vi "Result Info Schema Show FP.vi"(8 "error in (no error)":errorcluster, 10 "Test Log":refnum<vi>, 11 "Result Info in":refnum<class "Result Info.lvclass">) -> (0 "error out":errorcluster, 3 "Result Info out":refnum<class "Result Info.lvclass">)   [LabVIEW 2023]
uses:
  Result Info.lvclass
  D:/eDCU LTT/VT LTT Project/Source Code/Data Analysis/Subpanel-Abstract/Subpanel-Abstract.lvclass
  C:/Program Files/National Instruments/LabVIEW 2023/vi.lib/ActorFramework/Actor/Actor.lvclass
  D:/eDCU LTT/VT LTT Project/Source Code/Data Analysis/Result Info/Result Info/Result Info.lvclass
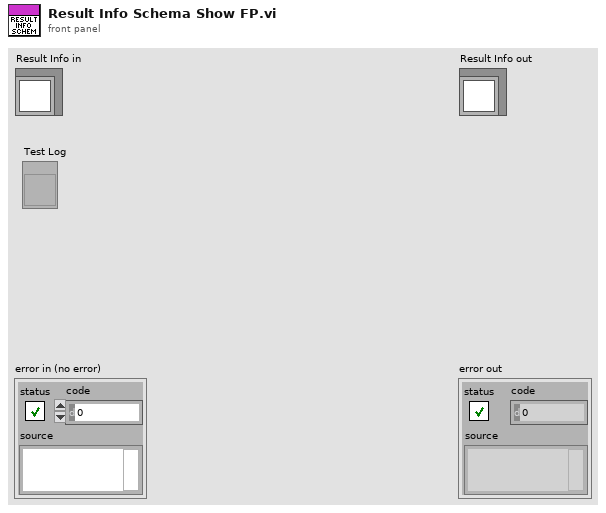
[diagram p1: front panel]
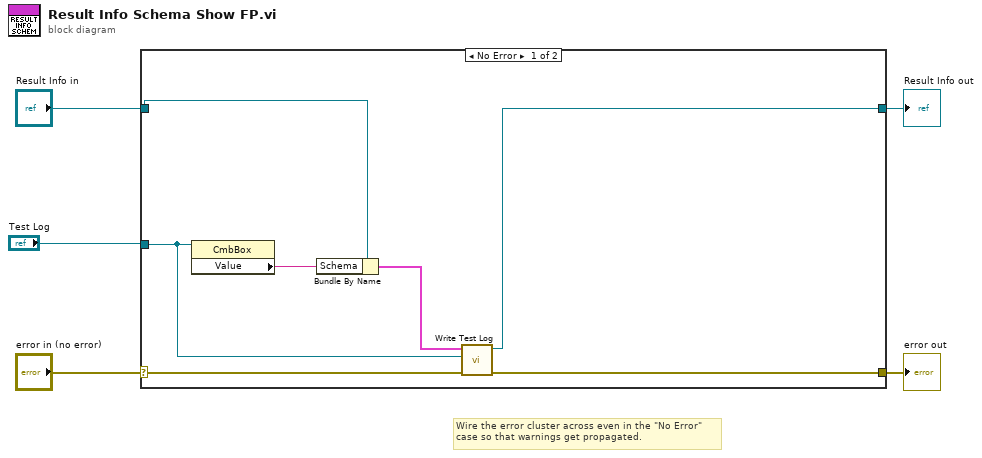
[diagram p0: block diagram]
diagram:
  # "Wire the error cluster across even in the \"No Error\"\ncase so that warnings get propagated."
  n1 = case shown="No Error" "error in (no error)" {
    selector: "error in (no error)" -> [w11 w14]
    tunnel: [w10 w14] -> w4
    tunnel: [w12 w13] -> w2
    tunnel: "Result Info in" -> [w8 w13]
    tunnel: "Test Log" -> [w9 _]
    frame No Error {
      n2 = property class="CmbBox"(reference=w9) -> ("Value"=w6:string)  [unwired: 1 in, 2 out]
      n3 = Bundle By Name(cluster=w8, "Schema"=w6) -> (w7:cluster{})
      n4 = call "Write Test Log.vi"("error in (no error)"=w11, "Test Log"=w9, "Result Info in"=w7) -> ("error out"=w10:errorcluster, "Result Info out"=w12:refnum<class "Result Info.lvclass">)  [unwired: 7 in]
    }
    frame Error {
    }
  }
  "error out" <- w4
  "Result Info out" <- w2
